vi "main - 副本.vi"() -> ()   [LabVIEW 2017]
uses:
  Ctrl/wave.ctl
  Ctrl/XYGraph.ctl
  <vilib>/Platform/TimedLoop/XDataNode/timing_clust.ctl
  <vilib>/Platform/TimedLoop/XDataNode/nitl_modes.ctl
  <vilib>/Platform/TimedLoop/XDataNode/wakeup.ctl
  <vilib>/Instr/_visa.llb/VISA Configure Serial Port (Instr).vi
  <vilib>/Platform/TimedLoop/XDataNode/XDataNode.xnode
  <vilib>/Platform/TimedLoop/XDataNode/XDNodeRunTimeDep.lvlib
panel:
  out "定时开始":bool=TRUE
  in  "XY缓存":cluster{dbl, dbl}[](array[cluster])
  in  "断开连接时使波形归零":bool
  out "误码":bool
  in  "图表点数":i32
  out "TX":dbl
  out "RX":u64
  in  "连接":bool
  out "串口状态":bool
  in  "波特率":u16(ring) items=["9600", "115200", "256000", "460800", "1000000"]
  in  "端口":string(combo)
  in  "界面切换":enum32{"测控", "后台状态"}(tab)
  in  "Y":enum16{"电流", "电压", "力", "位移", "电阻", "功率", "测试"}(ring)
  in  "X":enum16{"电流", "电压", "力", "位移", "电阻", "功率", "测试"}(ring)
  in  "复位系统":bool
  in  "测量倒计时 S":dbl format="%#.1f"
  out "能量 J":dbl format="%.4g"
  out "质量 g":dbl format="%.3g"
  out "功率 mW":dbl format="%.4g"
  out "电阻 R":dbl format="%.4g"
  in  "自动测量":bool
  out "湿度 %":dbl format="%.2g"
  out "温度 ℃":dbl format="%.2g"
  out "CPU %":u8
  out "位移 mm":dbl format="%.4g"
  out "力 mN":dbl format="%#.2g"
  out "电压 V":dbl format="%.4g"
  out "电流 mA":dbl format="%#.2g"
  in  "校准":bool
  in  "波形归零":bool
  in  "清空图表":bool
  out "持续时间 S":dbl format="%#.2g"
  out "系统时间":string
  in  "发送波形":bool
  out "波形图表":T1
  in  "波形选择":enum32{"斜坡", "正弦", "PWM波", "直流", "控制"}(tab)
  out "斜率k":dbl format="%#.2g"
  in  "通道D":enum16{"DA0", "DA1", "DA01", ""}(ring) caption="通道"
  in  "截距":dbl(slide) min=-5.0 max=5.0 step=0.01 scale=-4.0..4.0
  in  "斜率角":dbl(slide) step=0.01 scale=0.0..180.0
  in  "极值":dbl(slide) min=-5.0 max=5.0 step=0.01 scale=-4.0..4.0
  out "正弦频率":dbl caption="频率 f" format="%#.2g"
  in  "偏距":dbl(slide) min=-5.0 max=5.0 step=0.01 scale=-4.0..4.0
  in  "初相":dbl(slide) min=-6.5 max=6.5 step=0.01 scale=-7.0..7.0
  in  "振幅":dbl(slide) min=0.0 max=5.0 step=0.01 scale=0.0..4.0
  in  "正弦角频率":dbl(slide) caption="角频率" min=0.0 max=100.0 step=0.01 scale=0.0..65.0
  in  "通道S":enum16{"DA0", "DA1", "DA01", ""}(ring) caption="通道"
  in  "通道P":enum16{"DA0", "DA1", "DA01", ""}(ring) caption="通道"
  in  "占空比":dbl(slide) min=0.0 max=1.0 step=0.01 scale=0.0..1.0
  in  "PWM波频率":dbl(slide) caption="频率" min=0.0 max=1000.0 step=0.01 scale=0.0..50.0
  in  "低电压":dbl(slide) min=-5.0 max=5.0 step=0.01 scale=-4.0..4.0
  in  "高电压":dbl(slide) min=-5.0 max=5.0 step=0.01 scale=-4.0..4.0
  in  "DA0":dbl(slide) min=-5.0 max=5.0 step=0.01 scale=-4.0..4.0
  in  "DA1":dbl(slide) min=-5.0 max=5.0 step=0.01 scale=-4.0..4.0
  in  "DA01":dbl(slide) min=-5.0 max=5.0 step=0.01 scale=-4.0..4.0
  in  "控制方法":T2(ring)
  in  "闭环对象":enum16{"位移闭环", "功率闭环", "电流闭环", "力闭环"}(ring)
  in  "外环KP/Bind":dbl
  in  "KD":dbl min=0.0 max=5.0 step=1e-05
  in  "KI / LV":dbl
  in  "发送控制数据":bool
  in  "KP / HV":dbl
  in  "SetPoint":dbl
  in  "控制模式":bool
  in  "板子选择":bool
  out "XY图":T3
  in  "打开图表":bool
  in  "采样率 Hz":u16(ring) items=["10"=10, "20"=20, "50"=50, "100"=100]
  out "定时结束":dbl
  out "匹配剩余":string
  in  "发送区":string
  in  "换行":bool
  in  "send":bool
  in  "清空接收区":bool
  in  "接收间隔ms":u16(ring) items=["50"=50, "100"=100, "150"=150, "200"=200]
  out "实时采样率 Hz":i16
  in  "调试模式":bool
  out "接收区":string
  # "y=kt+b"
  # "y=Asin(ωt+φ)+k"
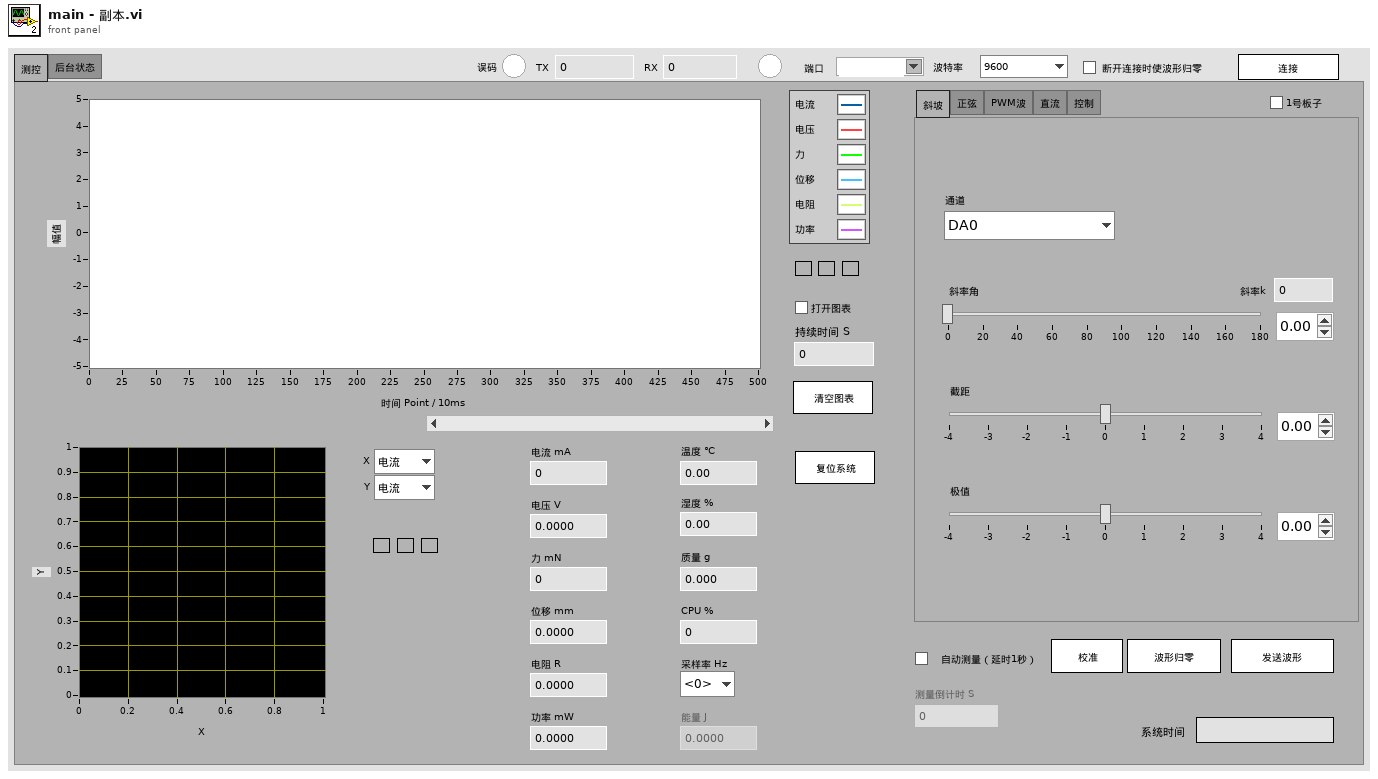
[diagram p1: front panel]
types:
  T1 = typedef "wave.ctl" = cluster{"电流":dbl, "电压":dbl, "力":dbl, "激光":dbl, "电阻":dbl, "功率":dbl}[]
  T2 = enum16{"PID控制", "BangBang控制", "串级PID控制", "自适应控制"}
  T3 = typedef "XYGraph.ctl" = cluster{"X":dbl, "Y":dbl}[]
  T4 = typedef "XDNodeRunTimeDep.lvlib/timing_clust.ctl" = cluster{"Expected End [f-1]":u64, "Actual End [f-1]":u64, "Finished Late? [f-1]":bool, "Expected End [i-1]":u64, "Actual End [i-1]":u64, "Finished Late? [i-1]":bool, "Expected Start [i]":u64, "Actual Start [i]":u64, "Expected Start [f]":u64, "Actual Start [f]":u64, "Source Name":string, "Structure Name":string, "Period":i64, "Deadline":i64, "Offset":i64, "Start":i64, "Priority":i32, "Timeout":i32, "Mode":T5, "Wakeup Reason":T6, "Error":errorcluster, "Source Type":string, "Secondary Source Type":string, "Global End Time":u64, "Global Start Time":u64, "Frame Duration":u64, "Iteration Duration":u64, "Assigned CPU":i32, "I/O Scan Engine Mode":u32}
  T5 = typedef "XDNodeRunTimeDep.lvlib/nitl_modes.ctl" = enum32{"No Change", "Process missed periods, maintain original phase", "Discard missed periods, maintain original phase", "Process missed periods, ignore original phase", "Discard missed periods, ignore original phase"}
  T6 = typedef "XDNodeRunTimeDep.lvlib/wakeup.ctl" = enum32{"Normal", "Aborted", "Asynchronous wakeup", "Timing source error", "Timed loop error", "Timeout"}
  T7 = cluster{"T0时间戳":dbl, "T1时间戳":dbl, "温度":dbl, "湿度":dbl, "CPU使用率":dbl}
  T8 = cluster{"电流":dbl, "电压":dbl, "力":dbl, "激光":dbl, "电阻":dbl, "功率":dbl}[]
  T9 = cluster{"电流":dbl, "电压":dbl, "力":dbl, "激光":dbl, "电阻":dbl, "功率":dbl}
  T10 = cluster{"X":enum16{"电流", "电压", "力", "位移", "电阻", "功率", "测试"}, "Y":enum16{"电流", "电压", "力", "位移", "电阻", "功率", "测试"}}
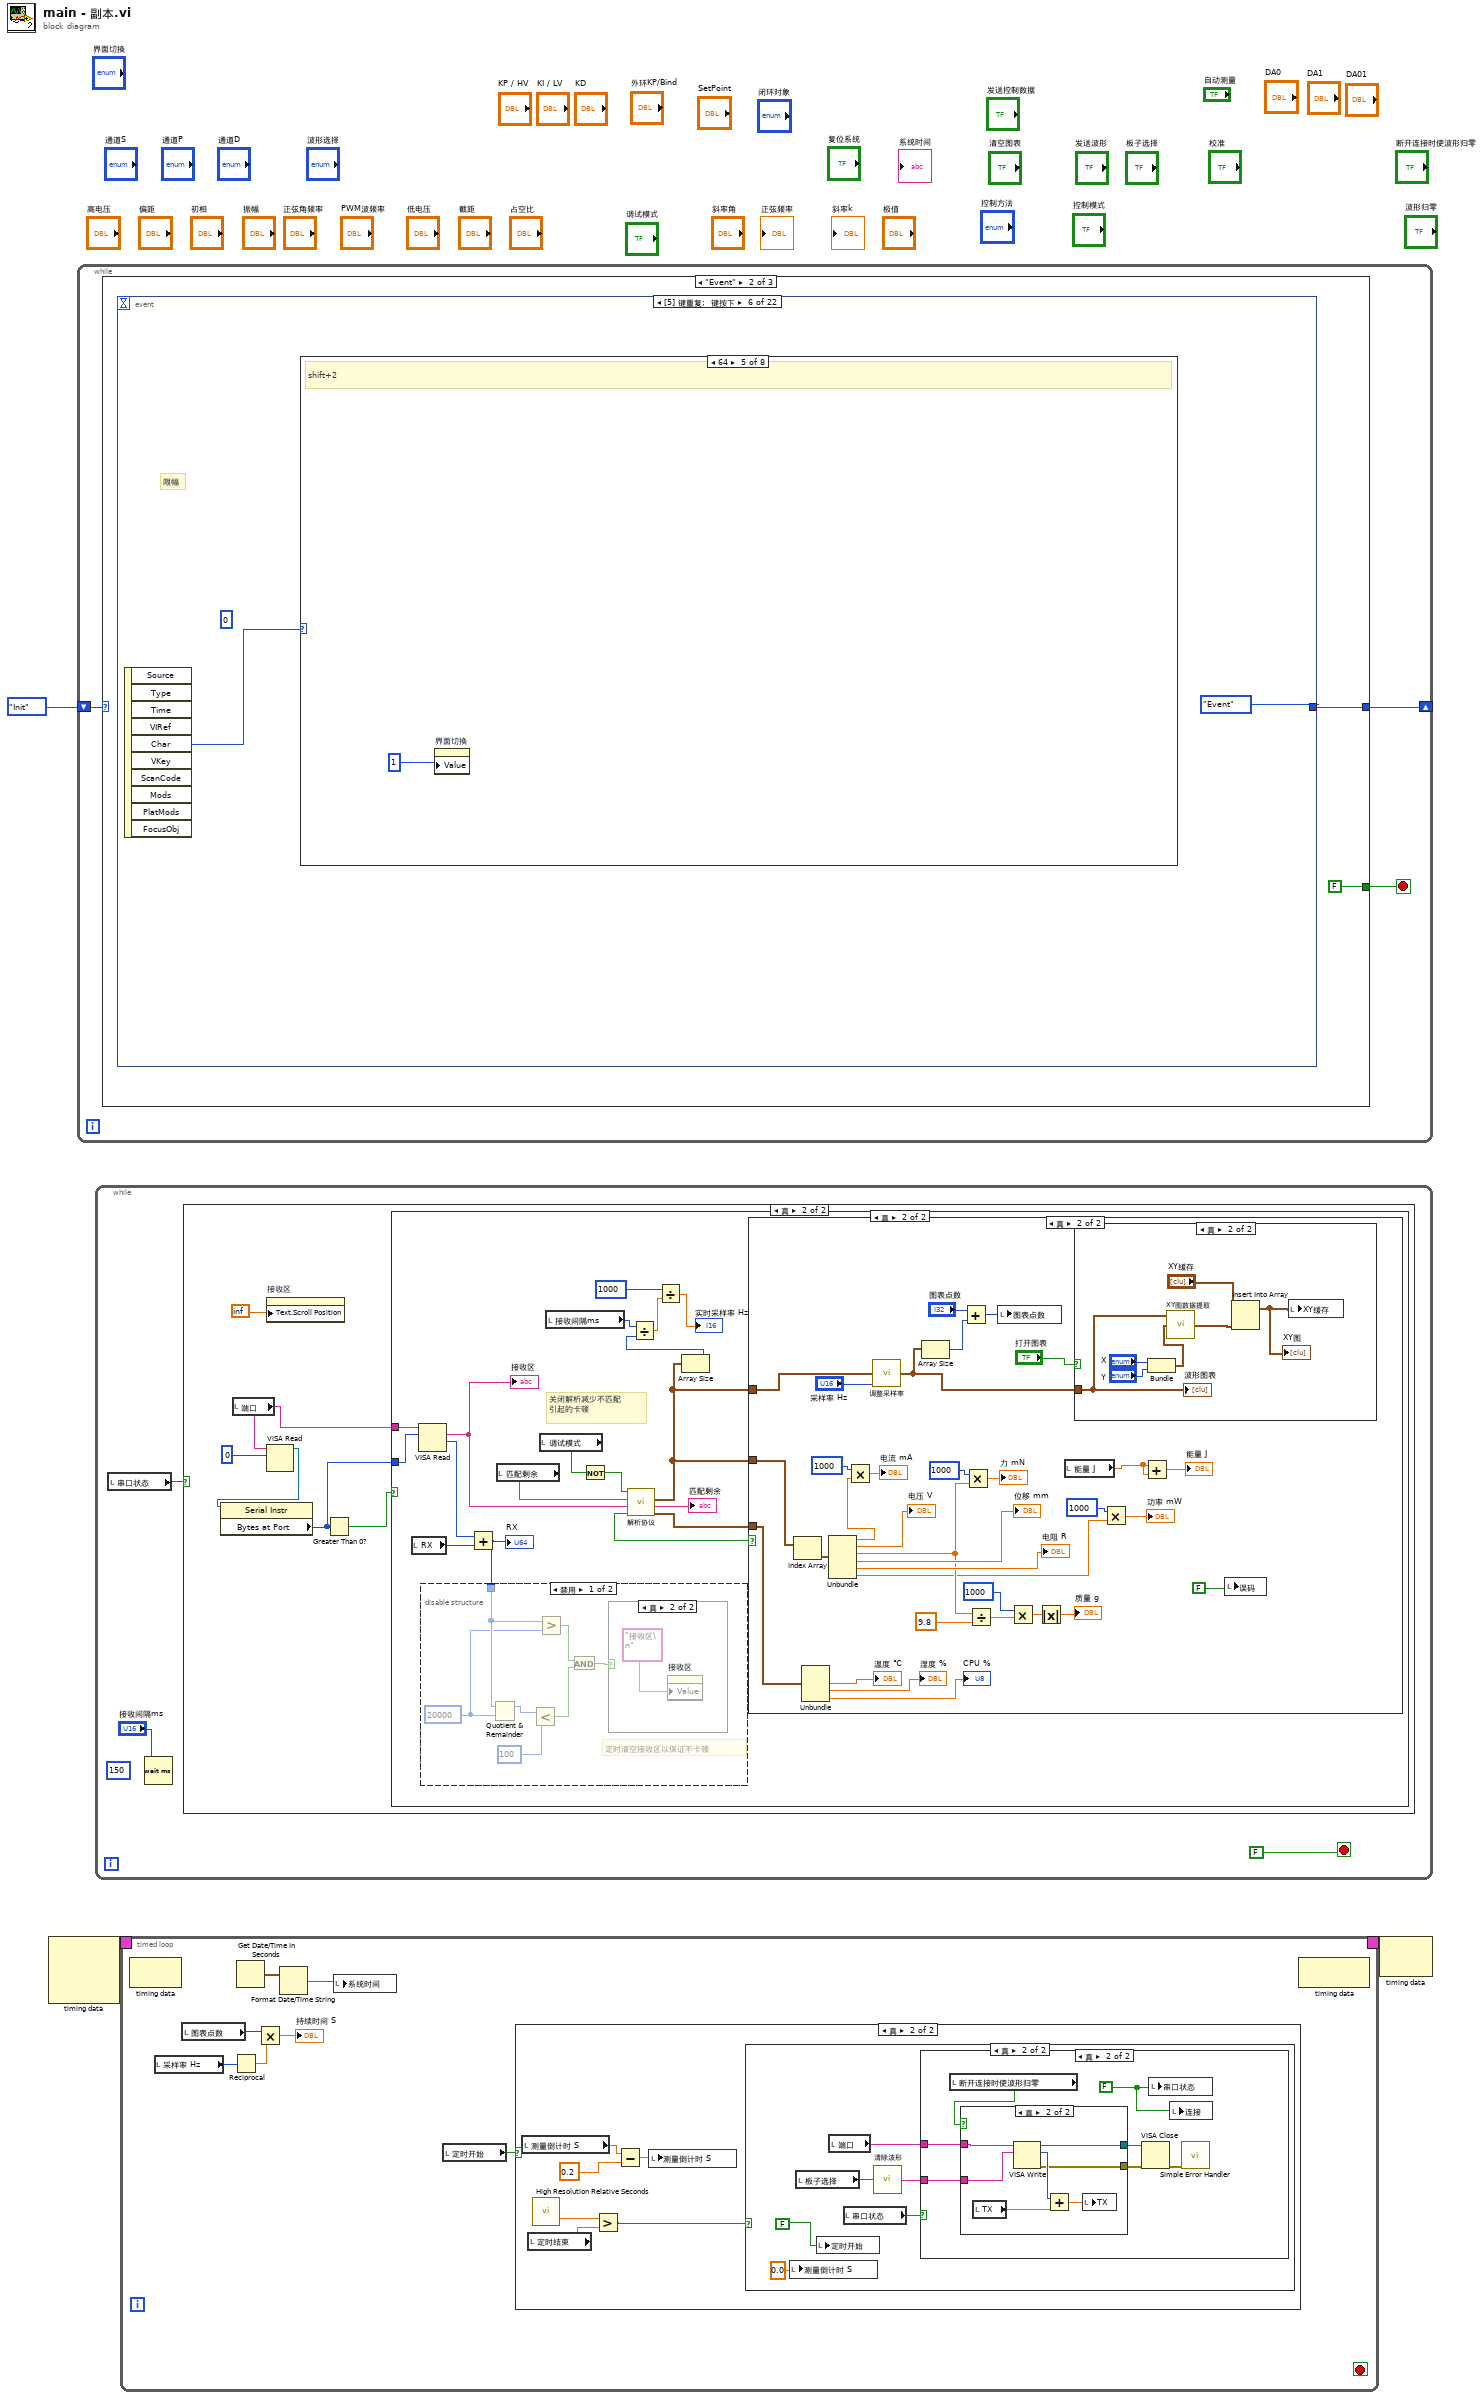
[diagram p0: block diagram]
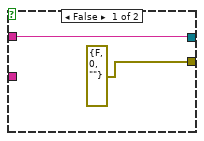
[diagram p5: hidden frame]
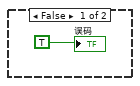
[diagram p10: hidden frame]
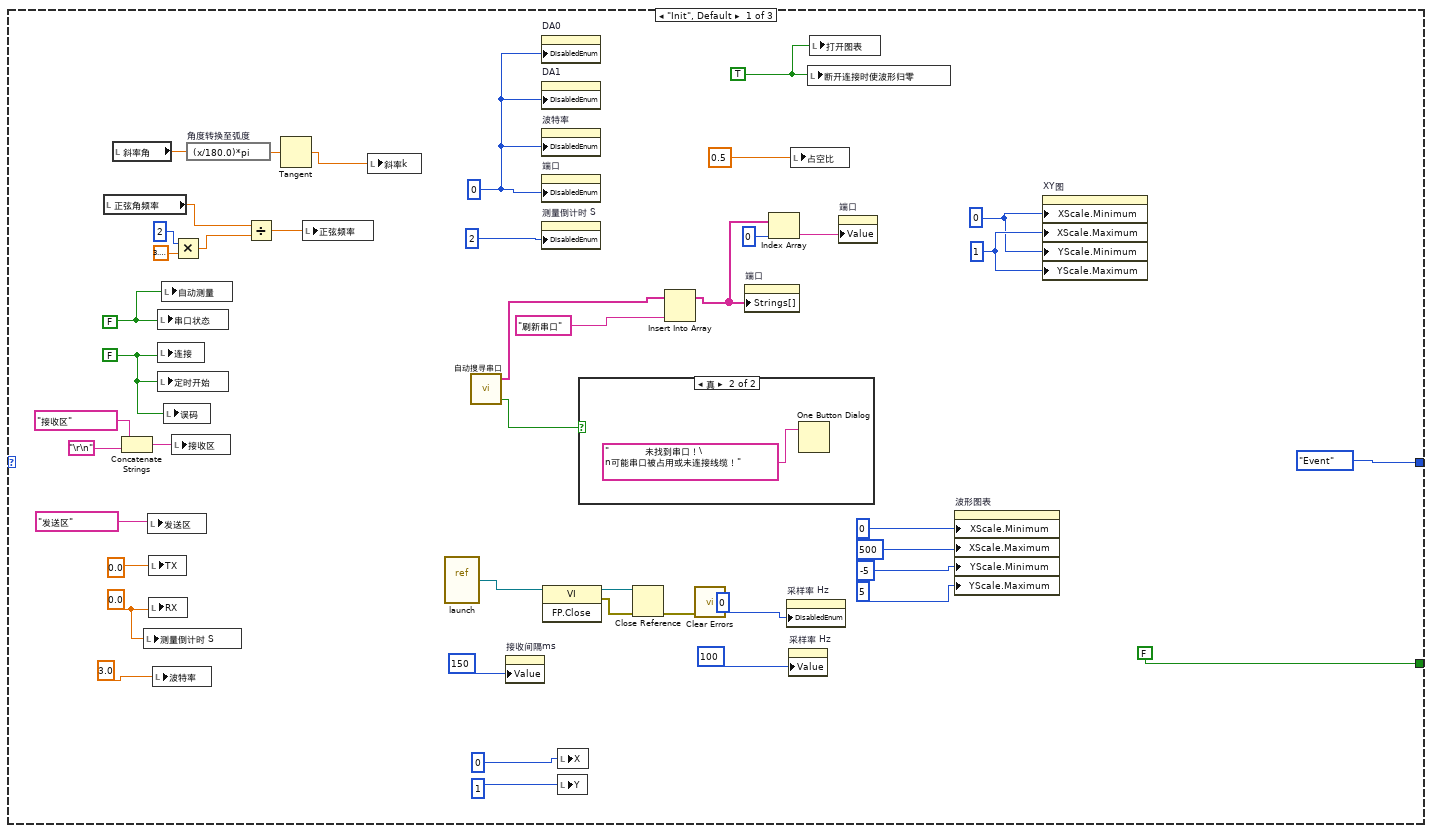
[diagram p12: hidden frame]
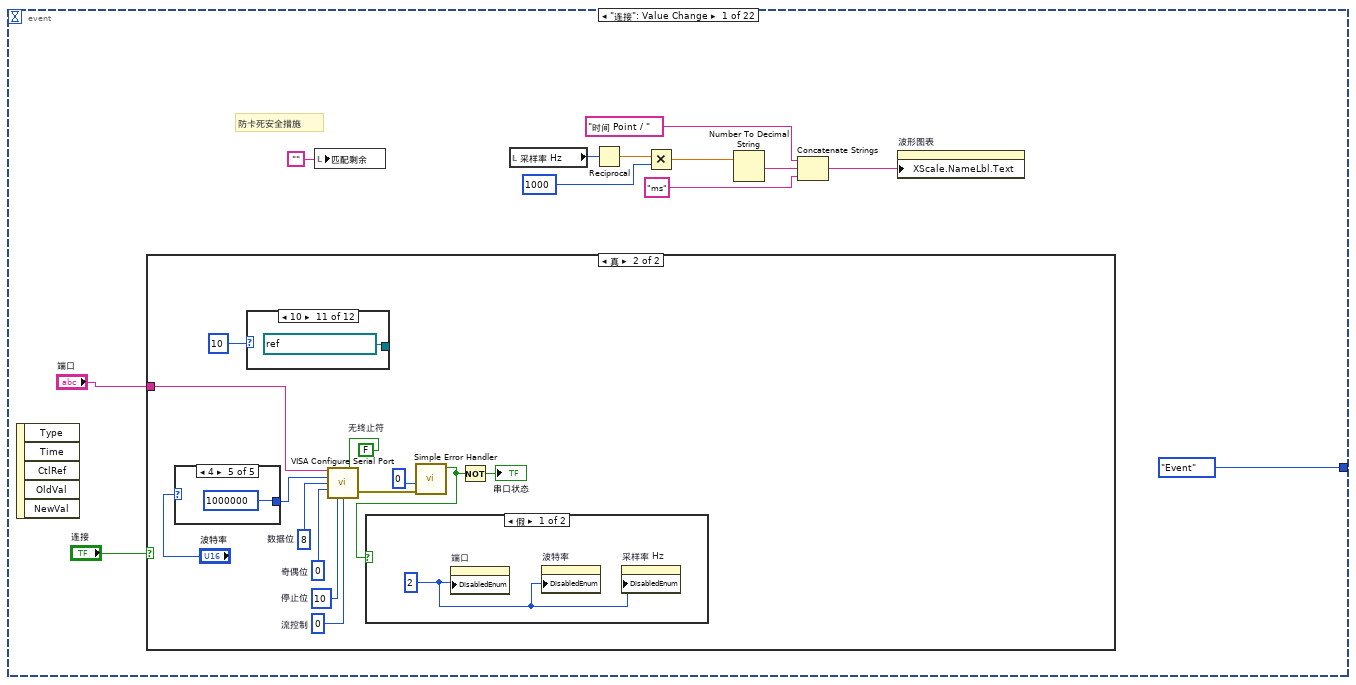
[diagram p14: hidden frame]
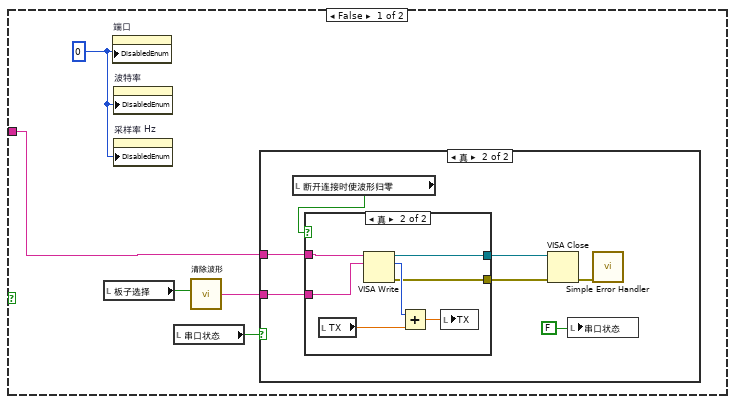
[diagram p15: hidden frame]
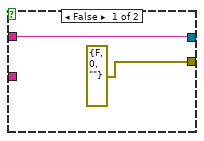
[diagram p17: hidden frame]
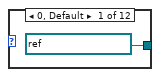
[diagram p18: hidden frame]
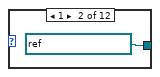
[diagram p19: hidden frame]
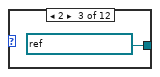
[diagram p20: hidden frame]
diagram:
  n1 = node-c288() -> (w2:T4)  [unwired: 3 in]
  n2 = while {
    shift-right: [w5] -> _
    shift-left: enum16{"Init", "Event", "Exit"}."Init" -> [w6]
    stop <- w4 stop-if-true
    n3 = case shown="\"Event\"" w6 {
      tunnel: [FALSE FALSE TRUE] -> w4
      tunnel: [enum16{"Init", "Event", "Exit"}."Event" w52 enum16{"Init", "Event", "Exit"}."Exit"] -> w5
      frame "Init", Default {
        w13 = 1
        w12 = 0
        w15 = TRUE
        w8 = 0
        w16 = 0.0 ("RX")
        w14 = FALSE
        w11 = FALSE
        n4 = local read "正弦角频率"() -> (w42:dbl)
        n5 = local read "斜率角"() -> (w46:dbl)
        n6 = Concatenate Strings("接收区", "\r\n") -> (w36:string)
        n7 = local write "测量倒计时 S"(w16) -> ()
        n8 = local write "发送区"("发送区") -> ()
        n9 = local write "TX"(0.0 ("TX")) -> ()
        n10 = local write "RX"(w16) -> ()
        n11 = local write "波特率"(3.0 ("RX")) -> ()
        n12 = local write "串口状态"(w14) -> ()
        n13 = local write "连接"(w11) -> ()
        n14 = local write "定时开始"(w11) -> ()
        n15 = local write "自动测量"(w14) -> ()
        n16 = local write "误码"(w11) -> ()
        n17 = local write "接收区"(w36) -> ()
        n18 = Multiply(x=2, y=3.141592653589793) -> (x*y=w41:dbl)
        n19 = expression code="(x/180.0)*pi" "角度转换至弧度"(w46) -> (w47:dbl)
        n20 = Divide(x=w42, y=w41) -> (x/y=w43:dbl)
        n21 = Tangent(1:w47) -> (0:w40:dbl)
        n22 = local write "正弦频率"(w43) -> ()
        n23 = local write "斜率k"(w40) -> ()
        n24 = vi-ref "launch.vi"() -> (w32:refnum<vi>)
        n25 = call "自动搜寻串口.vi"() -> ("找到的串口"=w34:string[], "有错误?"=w35:bool)  [unwired: 6 in, 1 out]
        n26 = property on="接收间隔ms" class="Ring (严格)"("Value"=150) -> ()  [unwired: 2 in, 2 out]
        n27 = property on="DA0" class="Slide (严格)"("DisabledEnum"=w8) -> ()  [unwired: 2 in, 2 out]
        n28 = property on="DA1" class="Slide (严格)"("DisabledEnum"=w8) -> ()  [unwired: 2 in, 2 out]
        n29 = property on="波特率" class="Ring (严格)"("DisabledEnum"=w8) -> ()  [unwired: 2 in, 2 out]
        n30 = property on="端口" class="CmbBox"("DisabledEnum"=w8) -> ()  [unwired: 2 in, 2 out]
        n31 = property on="测量倒计时 S" class="DigNum (严格)"("DisabledEnum"=2) -> ()  [unwired: 2 in, 2 out]
        n32 = invoke class="VI" method="FP.Close"(reference=w32) -> (reference out=w31:refnum<vi>, error out=w30:errorcluster)  [unwired: 2 in, 1 out]
        n33 = local write "X"(0) -> ()
        n34 = local write "Y"(1) -> ()
        n35 = case shown="真" w35 {
          frame False {
          }
          frame True {
            n36 = One Button Dialog(message="            未找到串口！\n可能串口被占用或未连接线缆！") -> ()  [unwired: 1 in, 1 out]
          }
        }
        n37 = Close Reference(reference=w31, error in (no error)=w30) -> (error out=w29:errorcluster)
        n38 = Insert Into Array(array=w34, new element="刷新串口") -> (w28:string[])  [unwired: 1 in]
        n39 = call <vilib>:"Clear Errors.vi"("error in (no error)"=w29) -> ()  [unwired: 5 in, 2 out]
        n40 = property on="端口" class="CmbBox"("Strings[]"=w28) -> ()  [unwired: 2 in, 2 out]
        n41 = Index Array(array=w28, index=0) -> (element=w26:string)
        n42 = property on="采样率 Hz" class="Ring (严格)"("DisabledEnum"=0) -> ()  [unwired: 2 in, 2 out]
        n43 = property on="采样率 Hz" class="Ring (严格)"("Value"=100) -> ()  [unwired: 2 in, 2 out]
        n44 = local write "占空比"(0.5 ("TX")) -> ()
        n45 = local write "断开连接时使波形归零"(w15) -> ()
        n46 = local write "打开图表"(w15) -> ()
        n47 = property on="端口" class="CmbBox"("Value"=w26) -> ()  [unwired: 2 in, 2 out]
        n48 = property on="波形图表" class="WFChart (严格)"("XScale.Minimum"=0, "XScale.Maximum"=500, "YScale.Minimum"=-5, "YScale.Maximum"=5) -> ()  [unwired: 2 in, 2 out]
        n49 = property on="XY图" class="XYGraph (严格)"("XScale.Minimum"=w12, "XScale.Maximum"=w13, "YScale.Minimum"=w12, "YScale.Maximum"=w13) -> ()  [unwired: 2 in, 2 out]
      }
      frame "Event" {
        n50 = event shown="[5] 键重复;  键按下" {
          selector: _ -> [_ _ _ _ _ _ _ _ _ _ _ _ _ _ _ _ _ _ _ _ _ _]
          dyn-events: _ -> [_ _ _ _ _ _ _ _ _ _ _ _ _ _ _ _ _ _ _ _ _ _]
          timeout: _ -> [_ _ _ _ _ _ _ _ _ _ _ _ _ _ _ _ _ _ _ _ _ _]
          tunnel: [enum16{"Init", "Event", "Exit"}."Event" enum16{"Init", "Event", "Exit"}."Event" enum16{"Init", "Event", "Exit"}."Event" enum16{"Init", "Event", "Exit"}."Event" enum16{"Init", "Event", "Exit"}."Event" enum16{"Init", "Event", "Exit"}."Event" enum16{"Init", "Event", "Exit"}."Event" enum16{"Init", "Event", "Exit"}."Event" enum16{"Init", "Event", "Exit"}."Event" enum16{"Init", "Event", "Exit"}."Event" enum16{"Init", "Event", "Exit"}."Event" enum16{"Init", "Event", "Exit"}."Event" enum16{"Init", "Event", "Exit"}."Event" enum16{"Init", "Event", "Exit"}."Event" enum16{"Init", "Event", "Exit"}."Event" enum16{"Init", "Event", "Exit"}."Event" enum16{"Init", "Event", "Exit"}."Event" enum16{"Init", "Event", "Exit"}."Event" enum16{"Init", "Event", "Exit"}."Event" enum16{"Init", "Event", "Exit"}."Event" enum16{"Init", "Event", "Exit"}."Event" enum16{"Init", "Event", "Exit"}."Event"] -> w52
          event "连接": Value Change {
            # "防卡死安全措施"
            n51 = event-data() -> ()  [unwired: 1 in, 5 out]
            n52 = case shown="真" "连接" {
              tunnel: "端口" -> [w66 w87]
              frame False {
                w70 = 0
                n53 = local read "板子选择"() -> (w69:bool)
                n54 = property on="端口" class="CmbBox"("DisabledEnum"=w70) -> ()  [unwired: 2 in, 2 out]
                n55 = property on="波特率" class="Ring (严格)"("DisabledEnum"=w70) -> ()  [unwired: 2 in, 2 out]
                n56 = property on="采样率 Hz" class="Ring (严格)"("DisabledEnum"=w70) -> ()  [unwired: 2 in, 2 out]
                n57 = local read "串口状态"() -> (w68:bool)
                n58 = call "清除波形.vi"("板子选择"=w69) -> ("输出字符串"=w67:string)
                n59 = case shown="真" w68 {
                  tunnel: w67 -> [_ w77]
                  tunnel: w66 -> [_ w72]
                  frame False {
                  }
                  frame True {
                    n60 = local read "断开连接时使波形归零"() -> (w71:bool)
                    n61 = case shown="真" w71 {
                      tunnel: w77 -> [_ w86]
                      tunnel: [w79 w82] -> w74
                      tunnel: [errorcluster {"status"=FALSE, "code"=0, "source"=""} ("错误常量") w81] -> w73
                      tunnel: w72 -> [w79 w80]
                      frame False {
                      }
                      frame True {
                        n62 = local read "TX"() -> (w84:dbl)
                        n63 = VISA Write(VISA resource name=w80, write buffer=w86) -> (VISA resource name out=w82:refnum<visa-resource-name>, return count=w85:u32, error out=w81:errorcluster)  [unwired: 1 in]
                        n64 = Add(x=w85, y=w84) -> (x+y=w83:dbl)
                        n65 = local write "TX"(w83) -> ()
                      }
                    }
                    n66 = VISA Close(VISA resource name=w74, error in (no error)=w73) -> (error out=w75:errorcluster)
                    n67 = local write "串口状态"(FALSE) -> ()
                    n68 = call <vilib>:"Simple Error Handler.vi"("error in (no error)"=w75) -> ()  [unwired: 4 in, 5 out]
                  }
                }
              }
              frame True {
                w90 = FALSE  # 无终止符
                w97 = u16 0  # 流控制
                w96 = u16 10  # 停止位
                w95 = u8 0  # 奇偶位
                w94 = u16 8  # 数据位
                n69 = case shown="4" "波特率" {
                  tunnel: [u32 9600 u32 115200 256000 460800 1000000] -> w93
                  frame 0 {
                  }
                  frame 1, Default {
                  }
                  frame 2 {
                  }
                  frame 3 {
                  }
                  frame 4 {
                  }
                }
                n70 = case shown="10" 10 {
                  tunnel: [refnum<visa-resource-name> "ASRL1::INSTR" ("VISA resource name") refnum<visa-resource-name> "ASRL2::INSTR" ("VISA resource name") refnum<visa-resource-name> "ASRL3::INSTR" ("VISA resource name") refnum<visa-resource-name> "ASRL4::INSTR" ("VISA resource name") refnum<visa-resource-name> "ASRL5::INSTR" ("VISA resource name") refnum<visa-resource-name> "ASRL6::INSTR" ("VISA resource name") refnum<visa-resource-name> "ASRL7::INSTR" ("VISA resource name") refnum<visa-resource-name> "ASRL8::INSTR" ("VISA resource name") refnum<visa-resource-name> "ASRL9::INSTR" ("VISA resource name") refnum<visa-resource-name> "ASRL10::INSTR" ("VISA resource name") refnum<visa-resource-name> "ASRL11::INSTR" ("VISA resource name") refnum<visa-resource-name> "ASRL12::INSTR" ("VISA resource name")] -> _
                  frame 0, Default {
                  }
                  frame 1 {
                  }
                  frame 2 {
                  }
                  frame 3 {
                  }
                  frame 4 {
                  }
                  frame 5 {
                  }
                  frame 6 {
                  }
                  frame 7 {
                  }
                  frame 8 {
                  }
                  frame 9 {
                  }
                  frame 10 {
                  }
                  frame 11 {
                  }
                }
                n71 = call-poly "VISA Configure Serial Port"("VISA resource name"=w87, "Enable Termination\nChar (T)"=w90, "baud rate (9600)"=w93, "data bits (8)"=w94, "parity (0:none)"=w95, "stop bits (10: 1 bit)"=w96, "flow control (0:none)"=w97) -> ("error out"=w98:errorcluster)  [unwired: 7 in, 1 out]
                n72 = call <vilib>:"Simple Error Handler.vi"("type of dialog (OK msg:1)"=0, "error in (no error)"=w98) -> ("error?"=w91:bool)  [unwired: 3 in, 4 out]
                n73 = case shown="假" w91 {
                  frame False {
                    w112 = 2
                    n74 = property on="端口" class="CmbBox"("DisabledEnum"=w112) -> ()  [unwired: 2 in, 2 out]
                    n75 = property on="波特率" class="Ring (严格)"("DisabledEnum"=w112) -> ()  [unwired: 2 in, 2 out]
                    n76 = property on="采样率 Hz" class="Ring (严格)"("DisabledEnum"=w112) -> ()  [unwired: 2 in, 2 out]
                  }
                  frame True {
                    n77 = One Button Dialog(message="串口不存在或已打开！\n请到“设备管理器”查看端口号COM！") -> ()  [unwired: 1 in, 1 out]
                    n78 = local write "连接"(FALSE) -> ()
                  }
                }
                n79 = Not(x=w91) -> (.not. x?=→"串口状态":bool)
              }
            }
            n80 = local write "匹配剩余"("") -> ()
            n81 = local read "采样率 Hz"() -> (w57:u16)
            n82 = Reciprocal(x=w57) -> (1/x=w56:dbl)
            n83 = Multiply(x=w56, y=1000) -> (x*y=w54:dbl)
            n84 = Number To Decimal String(number=w54) -> (decimal integer string=w61:string)  [unwired: 1 in]
            n85 = Concatenate Strings("时间 Point / ", w61, "ms") -> (w60:string)
            n86 = property on="波形图表" class="WFChart (严格)"("XScale.NameLbl.Text"=w60) -> ()  [unwired: 2 in, 2 out]
          }
          event "端口": Value Change {
            n87 = event-data() -> ("NewVal"=w123:string)  [unwired: 1 in, 5 out]
            n88 = Equal?(x=w123, y="刷新串口") -> (x = y?=w121:bool)
            n89 = case shown="真" w121 {
              frame False {
              }
              frame True {
                n90 = call "自动搜寻串口.vi"() -> ("找到的串口"=w127:string[], "有错误?"=w129:bool)  [unwired: 6 in, 1 out]
                n91 = case shown="真" w129 {
                  frame False {
                  }
                  frame True {
                    n92 = One Button Dialog(message="            未找到串口！\n可能串口被占用或未连接线缆！") -> ()  [unwired: 1 in, 1 out]
                  }
                }
                n93 = Insert Into Array(array=w127, new element="刷新串口") -> (w125:string[])  [unwired: 1 in]
                n94 = Index Array(array=w125, index=0) -> (element=w124:string)
                n95 = property on="端口" class="CmbBox"("Strings[]"=w125) -> ()  [unwired: 2 in, 2 out]
                n96 = property on="端口" class="CmbBox"("Value"=w124) -> ()  [unwired: 2 in, 2 out]
              }
            }
          }
          event "send": Mouse Down {
            n97 = event-data() -> ()  [unwired: 1 in, 7 out]
            n98 = local read "串口状态"() -> (w132:bool)
            n99 = case shown="真" w132 {
              frame False {
              }
              frame True {
                n100 = local read "端口"() -> (w133:string)
                n101 = case shown="真" "换行" {
                  tunnel: [_ "\r"] -> w141
                  tunnel: [_ "\n"] -> w140
                  frame False {
                  }
                  frame True {
                  }
                }
                n102 = Concatenate Strings("发送区", w141, w140) -> (w137:string)
                n103 = local read "TX"() -> (w136:dbl)
                n104 = VISA Write(VISA resource name=w133, write buffer=w137) -> (return count=w134:u32)  [unwired: 1 in, 2 out]
                n105 = Add(x=w134, y=w136) -> (x+y=→"TX":dbl)
              }
            }
          }
          event "清空接收区": Mouse Down {
            n106 = event-data() -> ()  [unwired: 1 in, 7 out]
            n107 = local write "接收区"("") -> ()
            n108 = local write "RX"(0.0 ("RX")) -> ()
            n109 = local write "TX"(0.0 ("TX")) -> ()
          }
          event Menu Selection (User) {
            n110 = event-data() -> ("ItemTag"=w148:string)  [unwired: 1 in, 5 out]
            n111 = case shown="\"电路板使用说明\"" w148 {
              frame "关于", Default {
                n112 = call "检查更新.vi"("超时ms"=3000.0) -> ("新版本号"=w152:string)  [unwired: 2 out]
                n113 = call "读取本地版本号.vi"() -> ("版本号"=w159:string)  [unwired: 6 in, 2 out]
                n114 = Concatenate Strings("最新版本号：", w152, "\r\n") -> (w151:string)
                n115 = Concatenate Strings("本地版本号：", w159, "\r\n") -> (w158:string)
                n116 = Concatenate Strings(w151, w158, "By YYH，IBSS，NUAA，NanJing，China") -> (w156:string)
                n117 = One Button Dialog(message=w156) -> ()  [unwired: 1 in, 1 out]
              }
              frame "存储曲线" {
                n118 = One Button Dialog(message="右键图表，点击“导出”即可。\n注意：只能导出显示范围数据，注意缩放") -> ()  [unwired: 1 in, 1 out]
              }
              frame "打开曲线" {
                n119 = One Button Dialog(message="暂不支持") -> ()  [unwired: 1 in, 1 out]
              }
              frame "数据协议" {
                n120 = call <vilib>:"Application Directory.vi"() -> ("Application Directory"=w166:path)
                n121 = call <vilib>:"System Exec.vi"("run minimized? (F)"=TRUE, "wait until completion? (T)"=FALSE, "working directory"=w166, "command line"="cmd /c start protocol.xlsx") -> ("error out"=w167:errorcluster)  [unwired: 4 in, 3 out]
                n122 = call <vilib>:"Simple Error Handler.vi"("error in (no error)"=w167) -> ()  [unwired: 4 in, 5 out]
              }
              frame "电路板使用说明" {
                n123 = One Button Dialog(message="电路板使用说明：\n\n灯光：\n常亮灯：电源指示灯\n闪烁灯：慢闪1次----程序运行正常\n            快闪2次----激光位移传感器通信失败\n            快闪4次----高负载警告\n            颜色--板子编号（蓝LED0、红LED1）\n\n按键：\nKEY键（位于边缘）：切换板子编号。\nRESET键（位于中间）：系统复位。\n\nUSB口：\n用于和电脑连接。\n\nCAN口：\n用于多电路板连接，CANH连CANH，CANL连CANL，并保证闪烁的灯颜色不一致。\n\nRJ11口（RS232）：\n用于和激光位移传感器KEYENCE LKGD500连接。") -> ()  [unwired: 1 in, 1 out]
              }
              frame "上位机使用说明" {
                n124 = One Button Dialog(message="上位机使用说明：\n\n鼠标悬停在部分控件上会自动出现说明提示。\n\nlaunch.exe：\n该文件为启动文件，用于检查软件更新，由于GitHub偶尔访问较慢，可进安装目录直接运行IPMC.exe（主程序文件）。\n\n连接：\n选择“端口号（刷新串口）”、“波特率（460800）”，点击“连接”--建立通信。\n\n误码：红灯亮起表示数据解析异常，请等待或重新连接。\n\n1/2号板子：\n选择要控制的电路板，1号板子--蓝灯闪烁，2号板子--红灯闪烁。\n\n快捷键：\n规划中...\n\n图表：\n1. 右键图表可以勾选自动缩放、存储曲线等功能；\n2. 导出曲线只导出可见范围内数据，要导出所有数据请先调整标尺；\n3. 图表缓存大小：1048576点；") -> ()  [unwired: 1 in, 1 out]
              }
            }
          }
          event Key Repeat; Key Down {
            (unwired) 0
            # "限幅"
            n125 = event-data() -> ("Char"=w170:i16)  [unwired: 1 in, 9 out]
            n126 = case "条件结构" shown="64" w170 {
              frame 0, Default {
              }
              frame 32 {
                # "空格"
                n127 = disable-structure shown="禁用" {
                  frame Disabled {
                    n128 = local read "板子选择"() -> (w173:bool)
                    n129 = local read "波形选择"() -> (w176:enum32{"斜坡", "正弦", "PWM波", "直流", "控制"})
                    n130 = Boolean To (0,1)(Boolean=w173) -> (0, 1=w172:i16)
                    n131 = case shown="\"斜坡\", 默认" w176 {
                      selector: w176 -> [w186 w199 w214 _]
                      tunnel: [w193 w202 w217 "\r\n"] -> w174
                      tunnel: w172 -> [w185 w198 w213 _]
                      frame "斜坡", Default {
                        w197 = 170
                        n132 = local read "通道D"() -> (w187:enum16{"DA0", "DA1", "DA01", ""})
                        n133 = local read "斜率k"() -> (w192:dbl)
                        n134 = local read "极值"() -> (w190:dbl)
                        n135 = local read "截距"() -> (w195:dbl)
                        n136 = call "浮点转字节数组.vi"("输入"=w190) -> ("数组，高字节在前"=w188:u8[])  [unwired: 3 in, 4 out]
                        n137 = call "浮点转字节数组.vi"("输入"=w192) -> ("数组，高字节在前"=w196:u8[])  [unwired: 3 in, 4 out]
                        n138 = call "浮点转字节数组.vi"("输入"=w195) -> ("数组，高字节在前"=w194:u8[])  [unwired: 3 in, 4 out]
                        n139 = Build Array (concatenate)(w197, w197, w185, w187, w186, w196, w194, w188, 0) -> (w191:u32[])
                        n140 = Byte Array To String(unsigned byte array=w191) -> (string=w193:string)
                        n141 = local write "发送区"(w193) -> ()
                      }
                      frame "正弦" {
                        w212 = 170
                        n142 = local read "通道S"() -> (w200:enum16{"DA0", "DA1", "DA01", ""})
                        n143 = local read "正弦角频率"() -> (w209:dbl)
                        n144 = local read "初相"() -> (w208:dbl)
                        n145 = local read "偏距"() -> (w204:dbl)
                        n146 = local read "振幅"() -> (w211:dbl)
                        n147 = call "浮点转字节数组.vi"("输入"=w211) -> ("数组，高字节在前"=w210:u8[])  [unwired: 3 in, 4 out]
                        n148 = call "浮点转字节数组.vi"("输入"=w209) -> ("数组，高字节在前"=w207:u8[])  [unwired: 3 in, 4 out]
                        n149 = call "浮点转字节数组.vi"("输入"=w208) -> ("数组，高字节在前"=w206:u8[])  [unwired: 3 in, 4 out]
                        n150 = call "浮点转字节数组.vi"("输入"=w204) -> ("数组，高字节在前"=w205:u8[])  [unwired: 3 in, 4 out]
                        n151 = Build Array (concatenate)(w212, w212, w198, w200, w199, w210, w207, w206, w205, 0) -> (w201:u32[])
                        n152 = Byte Array To String(unsigned byte array=w201) -> (string=w202:string)
                        n153 = local write "发送区"(w202) -> ()
                      }
                      frame "PWM波" {
                        w227 = 170
                        n154 = local read "通道P"() -> (w215:enum16{"DA0", "DA1", "DA01", ""})
                        n155 = local read "PWM波频率"() -> (w222:dbl)
                        n156 = local read "占空比"() -> (w220:dbl)
                        n157 = local read "高电压"() -> (w226:dbl)
                        n158 = local read "低电压"() -> (w224:dbl)
                        n159 = call "浮点转字节数组.vi"("输入"=w226) -> ("数组，高字节在前"=w225:u8[])  [unwired: 3 in, 4 out]
                        n160 = call "浮点转字节数组.vi"("输入"=w224) -> ("数组，高字节在前"=w223:u8[])  [unwired: 3 in, 4 out]
                        n161 = call "浮点转字节数组.vi"("输入"=w222) -> ("数组，高字节在前"=w221:u8[])  [unwired: 3 in, 4 out]
                        n162 = call "浮点转字节数组.vi"("输入"=w220) -> ("数组，高字节在前"=w219:u8[])  [unwired: 3 in, 4 out]
                        n163 = Build Array (concatenate)(w227, w227, w213, w215, w214, w225, w223, w221, w219, 0) -> (w216:u32[])
                        n164 = Byte Array To String(unsigned byte array=w216) -> (string=w217:string)
                        n165 = local write "发送区"(w217) -> ()
                      }
                      frame "直流" {
                      }
                    }
                    n166 = local read "串口状态"() -> (w175:bool)
                    n167 = case shown="真" w175 {
                      tunnel: w174 -> [_ w179]
                      frame False {
                        n168 = One Button Dialog(message="未连接平台！") -> ()  [unwired: 1 in, 1 out]
                      }
                      frame True {
                        n169 = local read "端口"() -> (w178:string)
                        n170 = Concatenate Strings(w179, "\r\n") -> (w184:string)
                        n171 = local read "TX"() -> (w182:dbl)
                        n172 = VISA Write(VISA resource name=w178, write buffer=w184) -> (return count=w183:u32)  [unwired: 1 in, 2 out]
                        n173 = Add(x=w183, y=w182) -> (x+y=w180:dbl)
                        n174 = local write "TX"(w180) -> ()
                      }
                    }
                  }
                  frame Enabled {
                  }
                }
              }
              frame 48 {
                # "字符0"
                n175 = disable-structure shown="禁用" {
                  frame Disabled {
                    w231 = 3  # 类型强制直流
                    w229 = 0.0
                    w232 = 2  # 通道
                    w233 = 170
                    n176 = local read "板子选择"() -> (w235:bool)
                    n177 = Boolean To (0,1)(Boolean=w235) -> (0, 1=w234:i16)
                    n178 = call "浮点转字节数组.vi"("输入"=w229) -> ("数组，高字节在前"=w236:u8[])  [unwired: 3 in, 4 out]
                    n179 = local write "DA0"(w229) -> ()
                    n180 = local write "DA1"(w229) -> ()
                    n181 = Build Array (concatenate)(w233, w233, w234, w232, w231, w236, w236, 0) -> (w239:i32[])
                    n182 = Byte Array To String(unsigned byte array=w239) -> (string=w238:string)
                    n183 = local write "发送区"(w238) -> ()
                    n184 = local read "串口状态"() -> (w237:bool)
                    n185 = case shown="真" w237 {
                      tunnel: w238 -> [_ w242]
                      frame False {
                        n186 = One Button Dialog(message="未连接平台！") -> ()  [unwired: 1 in, 1 out]
                      }
                      frame True {
                        n187 = local read "端口"() -> (w241:string)
                        n188 = Concatenate Strings(w242, "\r\n") -> (w247:string)
                        n189 = VISA Write(VISA resource name=w241, write buffer=w247) -> (return count=w246:u32)  [unwired: 1 in, 2 out]
                        n190 = local read "TX"() -> (w245:dbl)
                        n191 = Add(x=w246, y=w245) -> (x+y=w243:dbl)
                        n192 = local write "TX"(w243) -> ()
                      }
                    }
                  }
                  frame Enabled {
                  }
                }
              }
              frame 33 {
                # "shift+1"
                n193 = disable-structure shown="禁用" {
                  frame Disabled {
                    w256 = 1  # 通道
                    w261 = 170
                    n194 = local read "DA1"() -> (w264:dbl)
                    n195 = Add(x=-0.1, y=w264) -> (x+y=w262:dbl)
                    n196 = local write "DA1"(w262) -> ()
                    n197 = local read "板子选择"() -> (w255:bool)
                    n198 = local read "DA1"() -> (w252:dbl)
                    n199 = local read "DA0"() -> (w253:dbl)
                    n200 = Boolean To (0,1)(Boolean=w255) -> (0, 1=w254:i16)
                    n201 = call "浮点转字节数组.vi"("输入"=w253) -> ("数组，高字节在前"=w260:u8[])  [unwired: 3 in, 4 out]
                    n202 = call "浮点转字节数组.vi"("输入"=w252) -> ("数组，高字节在前"=w259:u8[])  [unwired: 3 in, 4 out]
                    n203 = Build Array (concatenate)(w261, w261, w254, w256, 3, w260, w259, 0) -> (w257:i32[])
                    n204 = local read "串口状态"() -> (w251:bool)
                    n205 = Byte Array To String(unsigned byte array=w257) -> (string=w250:string)
                    n206 = case shown="真" w251 {
                      tunnel: w250 -> [_ w269]
                      frame False {
                      }
                      frame True {
                        n207 = local read "端口"() -> (w271:string)
                        n208 = Concatenate Strings(w269, "\r\n") -> (w268:string)
                        n209 = local read "TX"() -> (w267:dbl)
                        n210 = VISA Write(VISA resource name=w271, write buffer=w268) -> (return count=w266:u32)  [unwired: 1 in, 2 out]
                        n211 = Add(x=w266, y=w267) -> (x+y=w265:dbl)
                        n212 = local write "TX"(w265) -> ()
                      }
                    }
                  }
                  frame Enabled {
                  }
                }
                n213 = property on="界面切换" class="TabCtl (严格)"("Value"=0) -> ()  [unwired: 2 in, 2 out]
              }
              frame 64 {
                # "shift+2"
                n214 = property on="界面切换" class="TabCtl (严格)"("Value"=1) -> ()  [unwired: 2 in, 2 out]
              }
              frame 51 {
                # "字符3"
                n215 = disable-structure shown="禁用" {
                  frame Disabled {
                    w279 = 1  # 通道
                    w281 = 170
                    n216 = local read "DA1"() -> (w288:dbl)
                    n217 = Add(x=0.1, y=w288) -> (x+y=w286:dbl)
                    n218 = local write "DA1"(w286) -> ()
                    n219 = local read "板子选择"() -> (w280:bool)
                    n220 = local read "DA0"() -> (w278:dbl)
                    n221 = local read "DA1"() -> (w277:dbl)
                    n222 = Boolean To (0,1)(Boolean=w280) -> (0, 1=w282:i16)
                    n223 = call "浮点转字节数组.vi"("输入"=w278) -> ("数组，高字节在前"=w285:u8[])  [unwired: 3 in, 4 out]
                    n224 = call "浮点转字节数组.vi"("输入"=w277) -> ("数组，高字节在前"=w284:u8[])  [unwired: 3 in, 4 out]
                    n225 = Build Array (concatenate)(w281, w281, w282, w279, 3, w285, w284, 0) -> (w275:i32[])
                    n226 = local read "串口状态"() -> (w276:bool)
                    n227 = Byte Array To String(unsigned byte array=w275) -> (string=w274:string)
                    n228 = case shown="真" w276 {
                      tunnel: w274 -> [_ w295]
                      frame False {
                      }
                      frame True {
                        n229 = local read "端口"() -> (w292:string)
                        n230 = Concatenate Strings(w295, "\r\n") -> (w293:string)
                        n231 = local read "TX"() -> (w290:dbl)
                        n232 = VISA Write(VISA resource name=w292, write buffer=w293) -> (return count=w289:u32)  [unwired: 1 in, 2 out]
                        n233 = Add(x=w289, y=w290) -> (x+y=w291:dbl)
                        n234 = local write "TX"(w291) -> ()
                      }
                    }
                  }
                  frame Enabled {
                  }
                }
              }
              frame 52 {
                # "字符4"
                n235 = disable-structure shown="禁用" {
                  frame Disabled {
                    w307 = 0  # 通道
                    w311 = 170
                    n236 = local read "DA0"() -> (w305:dbl)
                    n237 = Add(x=-0.1, y=w305) -> (x+y=w303:dbl)
                    n238 = local write "DA0"(w303) -> ()
                    n239 = local read "板子选择"() -> (w302:bool)
                    n240 = local read "DA1"() -> (w300:dbl)
                    n241 = local read "DA0"() -> (w301:dbl)
                    n242 = Boolean To (0,1)(Boolean=w302) -> (0, 1=w306:i16)
                    n243 = call "浮点转字节数组.vi"("输入"=w301) -> ("数组，高字节在前"=w310:u8[])  [unwired: 3 in, 4 out]
                    n244 = call "浮点转字节数组.vi"("输入"=w300) -> ("数组，高字节在前"=w309:u8[])  [unwired: 3 in, 4 out]
                    n245 = Build Array (concatenate)(w311, w311, w306, w307, 3, w310, w309, 0) -> (w299:i32[])
                    n246 = local read "串口状态"() -> (w297:bool)
                    n247 = Byte Array To String(unsigned byte array=w299) -> (string=w298:string)
                    n248 = case shown="真" w297 {
                      tunnel: w298 -> [_ w318]
                      frame False {
                      }
                      frame True {
                        n249 = local read "端口"() -> (w315:string)
                        n250 = Concatenate Strings(w318, "\r\n") -> (w316:string)
                        n251 = VISA Write(VISA resource name=w315, write buffer=w316) -> (return count=w314:u32)  [unwired: 1 in, 2 out]
                        n252 = local read "TX"() -> (w313:dbl)
                        n253 = Add(x=w314, y=w313) -> (x+y=w312:dbl)
                        n254 = local write "TX"(w312) -> ()
                      }
                    }
                  }
                  frame Enabled {
                  }
                }
              }
              frame 54 {
                # "字符6"
                n255 = disable-structure shown="禁用" {
                  frame Disabled {
                    w330 = 0  # 通道
                    w334 = 170
                    n256 = local read "DA0"() -> (w328:dbl)
                    n257 = Add(x=0.1, y=w328) -> (x+y=w327:dbl)
                    n258 = local write "DA0"(w327) -> ()
                    n259 = local read "板子选择"() -> (w325:bool)
                    n260 = local read "DA0"() -> (w324:dbl)
                    n261 = local read "DA0"() -> (w323:dbl)
                    n262 = Boolean To (0,1)(Boolean=w325) -> (0, 1=w329:i16)
                    n263 = call "浮点转字节数组.vi"("输入"=w324) -> ("数组，高字节在前"=w333:u8[])  [unwired: 3 in, 4 out]
                    n264 = call "浮点转字节数组.vi"("输入"=w323) -> ("数组，高字节在前"=w332:u8[])  [unwired: 3 in, 4 out]
                    n265 = Build Array (concatenate)(w334, w334, w329, w330, 3, w333, w332, 0) -> (w322:i32[])
                    n266 = local read "串口状态"() -> (w320:bool)
                    n267 = Byte Array To String(unsigned byte array=w322) -> (string=w321:string)
                    n268 = case shown="假" w320 {
                      tunnel: w321 -> [_ w341]
                      frame False {
                      }
                      frame True {
                        n269 = Concatenate Strings(w341, "\r\n") -> (w339:string)
                        n270 = local read "端口"() -> (w338:string)
                        n271 = VISA Write(VISA resource name=w338, write buffer=w339) -> (return count=w337:u32)  [unwired: 1 in, 2 out]
                        n272 = local read "TX"() -> (w336:dbl)
                        n273 = Add(x=w337, y=w336) -> (x+y=w335:dbl)
                        n274 = local write "TX"(w335) -> ()
                      }
                    }
                  }
                  frame Enabled {
                  }
                }
              }
            }
          }
          event "清空图表": Mouse Up {
            n275 = event-data() -> ()  [unwired: 1 in, 8 out]
            n276 = Two Button Dialog(message="确认清空图表吗？") -> (T button?=w342:bool)  [unwired: 2 in]
            n277 = case shown="真" w342 {
              frame False {
              }
              frame True {
                w350 = 1
                w351 = 0
                w352 = cluster{dbl, dbl}[] []
                w349 = 0
                n278 = local write "图表点数"(w349) -> ()
                n279 = property on="波形图表" class="WFChart (严格)"("XScale.Minimum"=w349, "XScale.Maximum"=500, "YScale.Minimum"=-5, "YScale.Maximum"=5) -> ()  [unwired: 2 in, 2 out]
                n280 = local write "XY缓存"(w352) -> ()
                n281 = property on="XY图" class="XYGraph (严格)"("Value"=w352) -> ()  [unwired: 2 in, 2 out]
                n282 = property on="波形图表" class="WFChart (严格)"("History Data"=cluster{dbl, dbl, dbl, dbl, dbl, dbl}[] []) -> ()  [unwired: 2 in, 2 out]
                n283 = property on="XY图" class="XYGraph (严格)"("XScale.Minimum"=w351, "XScale.Maximum"=w350, "YScale.Minimum"=w351, "YScale.Maximum"=w350) -> ()  [unwired: 2 in, 2 out]
              }
            }
          }
          event "X", "Y": Value Change {
            w353 = cluster{dbl, dbl}[] []
            n284 = event-data() -> ()  [unwired: 1 in, 6 out]
            n285 = local write "XY缓存"(w353) -> ()
            n286 = property on="XY图" class="XYGraph (严格)"("Value"=w353) -> ()  [unwired: 2 in, 2 out]
          }
          event "校准": Mouse Up {
            w355 = u16 170 items=["0xAA"=170, "CH0"=0, "CH1"=1, "CH01"=2, "CARLIB"=85, "SWITCH"=86, "CONTROL"=87]
            w356 = u16 85 items=["0xAA"=170, "CH0"=0, "CH1"=1, "CH01"=2, "CARLIB"=85, "SWITCH"=86, "CONTROL"=87]
            w359 = "\r\n"
            n287 = event-data() -> ()  [unwired: 1 in, 8 out]
            n288 = local read "板子选择"() -> (w365:bool)
            n289 = Boolean To (0,1)(Boolean=w365) -> (0, 1=w364:i16)
            n290 = Build Array(w355, w355, w364, w356, w356) -> (w363:u16[])
            n291 = Byte Array To String(unsigned byte array=w363) -> (string=w362:string)
            n292 = Concatenate Strings(w362, "CARLIB", w359, w359) -> (w357:string)
            n293 = local read "串口状态"() -> (w361:bool)
            n294 = local write "发送区"(w357) -> ()
            n295 = case shown="真" w361 {
              tunnel: w357 -> [_ w366]
              frame False {
              }
              frame True {
                n296 = local read "端口"() -> (w368:string)
                n297 = local read "TX"() -> (w369:dbl)
                n298 = VISA Write(VISA resource name=w368, write buffer=w366) -> (return count=w367:u32)  [unwired: 1 in, 2 out]
                n299 = Add(x=w367, y=w369) -> (x+y=w370:dbl)
                n300 = local write "TX"(w370) -> ()
              }
            }
          }
          event "波形归零": Mouse Up; "控制模式", "调试模式": Value Change {
            w381 = u16 170 items=["0xAA"=170, "CH0"=0, "CH1"=1, "CH01"=2, "CARLIB"=85, "SWITCH"=86, "CONTROL"=87]
            w380 = u16 86 items=["0xAA"=170, "CH0"=0, "CH1"=1, "CH01"=2, "CARLIB"=85, "SWITCH"=86, "CONTROL"=87]
            n301 = event-data() -> ()  [unwired: 1 in, 4 out]
            n302 = local read "控制模式"() -> (w379:bool)
            n303 = local read "板子选择"() -> (w383:bool)
            n304 = case shown="假" w379 {
              tunnel: 0 -> [w394 w398]
              tunnel: [w393 w396] -> w376
              frame False {
                n305 = And(x=127, y=w394) -> (x .and. y?=w393:i32)
              }
              frame True {
                n306 = Or(x=128, y=w398) -> (x .or. y?=w396:i32)
              }
            }
            n307 = Boolean To (0,1)(Boolean=w383) -> (0, 1=w382:i16)
            n308 = local read "串口状态"() -> (w385:bool)
            n309 = call "清除波形.vi"() -> ()  [unwired: 1 in, 1 out]
            n310 = local read "调试模式"() -> (w377:bool)
            n311 = case shown="真" w377 {
              tunnel: w376 -> [w388 w392]
              tunnel: [w387 w390] -> w375
              frame False {
                n312 = And(x=191, y=w388) -> (x .and. y?=w387:i32)
              }
              frame True {
                n313 = Or(x=64, y=w392) -> (x .or. y?=w390:i32)
              }
            }
            n314 = Or(x=32, y=w375) -> (x .or. y?=w373:i32)
            n315 = Build Array(w381, w381, w382, w380, w380, w373, 0) -> (w384:i32[])
            n316 = Byte Array To String(unsigned byte array=w384) -> (string=w371:string)
            n317 = case shown="真" w385 {
              tunnel: w371 -> [_ w401]
              frame False {
                n318 = One Button Dialog(message="未连接平台！") -> ()  [unwired: 1 in, 1 out]
              }
              frame True {
                w400 = 0.0
                n319 = local read "端口"() -> (w402:string)
                n320 = local read "TX"() -> (w404:dbl)
                n321 = VISA Write(VISA resource name=w402, write buffer=w401) -> (return count=w405:u32)  [unwired: 1 in, 2 out]
                n322 = Add(x=w405, y=w404) -> (x+y=w403:dbl)
                n323 = local write "DA0"(w400) -> ()
                n324 = local write "DA1"(w400) -> ()
                n325 = local write "DA01"(w400) -> ()
                n326 = local write "TX"(w403) -> ()
              }
            }
          }
          event "复位系统": Mouse Up {
            n327 = event-data() -> ()  [unwired: 1 in, 8 out]
            n328 = Two Button Dialog(message="确认复位电路板吗？") -> (T button?=w407:bool)  [unwired: 2 in]
            n329 = case shown="真" w407 {
              frame False {
              }
              frame True {
                w416 = u16 170 items=["0xAA"=170, "CH0"=0, "CH1"=1, "CH01"=2, "CARLIB"=85, "SWITCH"=86, "CONTROL"=87]
                w417 = u16 86 items=["0xAA"=170, "CH0"=0, "CH1"=1, "CH01"=2, "CARLIB"=85, "SWITCH"=86, "CONTROL"=87]
                n330 = local read "板子选择"() -> (w415:bool)
                n331 = Boolean To (0,1)(Boolean=w415) -> (0, 1=w414:i16)
                n332 = local read "串口状态"() -> (w411:bool)
                n333 = Build Array(w416, w416, w414, w417, w417, 8, 0) -> (w412:i32[])
                n334 = Byte Array To String(unsigned byte array=w412) -> (string=w410:string)
                n335 = case shown="真" w411 {
                  tunnel: w410 -> [_ w419]
                  frame False {
                    n336 = One Button Dialog(message="未连接平台！") -> ()  [unwired: 1 in, 1 out]
                  }
                  frame True {
                    n337 = local read "端口"() -> (w423:string)
                    n338 = local read "TX"() -> (w422:dbl)
                    n339 = VISA Write(VISA resource name=w423, write buffer=w419) -> (return count=w420:u32)  [unwired: 1 in, 2 out]
                    n340 = Add(x=w420, y=w422) -> (x+y=w421:dbl)
                    n341 = local write "TX"(w421) -> ()
                  }
                }
              }
            }
          }
          event "发送波形": Mouse Up {
            n342 = event-data() -> ()  [unwired: 1 in, 8 out]
            n343 = flat-sequence {
              frame #0 {
                n344 = local read "自动测量"() -> (w425:bool)
                n345 = case shown="真" w425 {
                  frame False {
                  }
                  frame True {
                    w430 = 1
                    w431 = 0
                    w429 = 0
                    w435 = cluster{dbl, dbl}[] []
                    n346 = local write "图表点数"(w429) -> ()
                    n347 = Greater Than 0?(x="测量倒计时 S") -> (x > 0?=w432:bool)
                    n348 = property on="波形图表" class="WFChart (严格)"("XScale.Minimum"=w429, "XScale.Maximum"=500, "YScale.Minimum"=-5, "YScale.Maximum"=5) -> ()  [unwired: 2 in, 2 out]
                    n349 = case shown="真" w432 {
                      frame False {
                      }
                      frame True {
                        n350 = local read "测量倒计时 S"() -> (w440:dbl)
                        n351 = call <vilib>:"High Resolution Relative Seconds.vi"() -> ("relative seconds"=w441:dbl)
                        n352 = Add(x=w441, y=w440) -> (x+y=→"定时结束":dbl)
                        "定时开始" <- TRUE
                      }
                    }
                    n353 = local write "图表点数"(0.0) -> ()
                    n354 = local write "XY缓存"(w435) -> ()
                    n355 = property on="波形图表" class="WFChart (严格)"("History Data"=cluster{dbl, dbl, dbl, dbl, dbl, dbl}[] []) -> ()  [unwired: 2 in, 2 out]
                    n356 = Wait (ms)(milliseconds to wait=1000) -> ()  [unwired: 1 out]
                    n357 = property on="XY图" class="XYGraph (严格)"("XScale.Minimum"=w431, "XScale.Maximum"=w430, "YScale.Minimum"=w431, "YScale.Maximum"=w430) -> ()  [unwired: 2 in, 2 out]
                    n358 = property on="XY图" class="XYGraph (严格)"("Value"=w435) -> ()  [unwired: 2 in, 2 out]
                  }
                }
              }
              frame #1 {
                n359 = local read "板子选择"() -> (w445:bool)
                n360 = local read "波形选择"() -> (w446:enum32{"斜坡", "正弦", "PWM波", "直流", "控制"})
                n361 = Boolean To (0,1)(Boolean=w445) -> (0, 1=w444:i16)
                n362 = case shown="\"斜坡\", 默认" w446 {
                  selector: w446 -> [w456 w469 w484 w500]
                  tunnel: [w463 w472 w487 w499] -> w442
                  tunnel: w444 -> [w455 w468 w483 w501]
                  frame "斜坡", Default {
                    w467 = 170
                    n363 = local read "通道D"() -> (w457:enum16{"DA0", "DA1", "DA01", ""})
                    n364 = local read "斜率k"() -> (w462:dbl)
                    n365 = local read "极值"() -> (w460:dbl)
                    n366 = local read "截距"() -> (w465:dbl)
                    n367 = call "浮点转字节数组.vi"("输入"=w460) -> ("数组，高字节在前"=w458:u8[])  [unwired: 3 in, 4 out]
                    n368 = call "浮点转字节数组.vi"("输入"=w462) -> ("数组，高字节在前"=w466:u8[])  [unwired: 3 in, 4 out]
                    n369 = call "浮点转字节数组.vi"("输入"=w465) -> ("数组，高字节在前"=w464:u8[])  [unwired: 3 in, 4 out]
                    n370 = Build Array (concatenate)(w467, w467, w455, w457, w456, w466, w464, w458, 0) -> (w461:u32[])
                    n371 = Byte Array To String(unsigned byte array=w461) -> (string=w463:string)
                    n372 = local write "发送区"(w463) -> ()
                  }
                  frame "正弦" {
                    w482 = 170
                    n373 = local read "通道S"() -> (w470:enum16{"DA0", "DA1", "DA01", ""})
                    n374 = local read "正弦角频率"() -> (w479:dbl)
                    n375 = local read "初相"() -> (w478:dbl)
                    n376 = local read "偏距"() -> (w474:dbl)
                    n377 = local read "振幅"() -> (w481:dbl)
                    n378 = call "浮点转字节数组.vi"("输入"=w481) -> ("数组，高字节在前"=w480:u8[])  [unwired: 3 in, 4 out]
                    n379 = call "浮点转字节数组.vi"("输入"=w479) -> ("数组，高字节在前"=w477:u8[])  [unwired: 3 in, 4 out]
                    n380 = call "浮点转字节数组.vi"("输入"=w478) -> ("数组，高字节在前"=w476:u8[])  [unwired: 3 in, 4 out]
                    n381 = call "浮点转字节数组.vi"("输入"=w474) -> ("数组，高字节在前"=w475:u8[])  [unwired: 3 in, 4 out]
                    n382 = Build Array (concatenate)(w482, w482, w468, w470, w469, w480, w477, w476, w475, 0) -> (w471:u32[])
                    n383 = Byte Array To String(unsigned byte array=w471) -> (string=w472:string)
                    n384 = local write "发送区"(w472) -> ()
                  }
                  frame "PWM波" {
                    w497 = 170
                    n385 = local read "通道P"() -> (w485:enum16{"DA0", "DA1", "DA01", ""})
                    n386 = local read "PWM波频率"() -> (w492:dbl)
                    n387 = local read "占空比"() -> (w490:dbl)
                    n388 = local read "高电压"() -> (w496:dbl)
                    n389 = local read "低电压"() -> (w494:dbl)
                    n390 = call "浮点转字节数组.vi"("输入"=w496) -> ("数组，高字节在前"=w495:u8[])  [unwired: 3 in, 4 out]
                    n391 = call "浮点转字节数组.vi"("输入"=w494) -> ("数组，高字节在前"=w493:u8[])  [unwired: 3 in, 4 out]
                    n392 = call "浮点转字节数组.vi"("输入"=w492) -> ("数组，高字节在前"=w491:u8[])  [unwired: 3 in, 4 out]
                    n393 = call "浮点转字节数组.vi"("输入"=w490) -> ("数组，高字节在前"=w489:u8[])  [unwired: 3 in, 4 out]
                    n394 = Build Array (concatenate)(w497, w497, w483, w485, w484, w495, w493, w491, w489, 0) -> (w486:u32[])
                    n395 = Byte Array To String(unsigned byte array=w486) -> (string=w487:string)
                    n396 = local write "发送区"(w487) -> ()
                  }
                  frame "直流" {
                    n397 = local read "自动测量"() -> (w498:bool)
                    n398 = case shown="真" w498 {
                      tunnel: w501 -> [_ w510]
                      tunnel: w500 -> [_ w507]
                      tunnel: ["\r\n" w503] -> w499
                      frame False {
                      }
                      frame True {
                        w508 = 2  # 通道
                        w509 = 170
                        n399 = local read "DA01"() -> (w506:dbl)
                        n400 = local read "DA01"() -> (w505:dbl)
                        n401 = call "浮点转字节数组.vi"("输入"=w506) -> ("数组，高字节在前"=w513:u8[])  [unwired: 3 in, 4 out]
                        n402 = call "浮点转字节数组.vi"("输入"=w505) -> ("数组，高字节在前"=w512:u8[])  [unwired: 3 in, 4 out]
                        n403 = Build Array (concatenate)(w509, w509, w510, w508, w507, w513, w512, 0) -> (w504:u32[])
                        n404 = Byte Array To String(unsigned byte array=w504) -> (string=w503:string)
                      }
                    }
                    n405 = local write "发送区"(w499) -> ()
                  }
                }
                n406 = local read "串口状态"() -> (w443:bool)
                n407 = case shown="真" w443 {
                  tunnel: w442 -> [_ w448]
                  frame False {
                    n408 = One Button Dialog(message="未连接平台！") -> ()  [unwired: 1 in, 1 out]
                  }
                  frame True {
                    n409 = local read "端口"() -> (w449:string)
                    n410 = Concatenate Strings(w448, "\r\n") -> (w454:string)
                    n411 = local read "TX"() -> (w452:dbl)
                    n412 = VISA Write(VISA resource name=w449, write buffer=w454) -> (return count=w453:u32)  [unwired: 1 in, 2 out]
                    n413 = Add(x=w453, y=w452) -> (x+y=w450:dbl)
                    n414 = local write "TX"(w450) -> ()
                  }
                }
              }
            }
          }
          event "自动测量": Value Change {
            n415 = event-data() -> ("NewVal"=w514:bool)  [unwired: 1 in, 5 out]
            n416 = case shown="真" w514 {
              frame False {
                w516 = 0
                n417 = property on="DA0" class="Slide (严格)"("DisabledEnum"=w516) -> ()  [unwired: 2 in, 2 out]
                n418 = property on="DA1" class="Slide (严格)"("DisabledEnum"=w516) -> ()  [unwired: 2 in, 2 out]
                n419 = property on="测量倒计时 S" class="DigNum (严格)"("DisabledEnum"=2) -> ()  [unwired: 2 in, 2 out]
              }
              frame True {
                w518 = 2
                n420 = property on="测量倒计时 S" class="DigNum (严格)"("DisabledEnum"=0) -> ()  [unwired: 2 in, 2 out]
                n421 = property on="DA0" class="Slide (严格)"("DisabledEnum"=w518) -> ()  [unwired: 2 in, 2 out]
                n422 = property on="DA1" class="Slide (严格)"("DisabledEnum"=w518) -> ()  [unwired: 2 in, 2 out]
              }
            }
          }
          event "断开连接时使波形归零": Value Change {
            n423 = event-data() -> ("NewVal"=w521:bool)  [unwired: 1 in, 5 out]
            n424 = case shown="假" w521 {
              frame False {
                n425 = One Button Dialog(message="断开连接后，平台将继续输出波形，但无法继续采集数据！") -> ()  [unwired: 1 in, 1 out]
              }
              frame True {
              }
            }
          }
          event "DA0": Value Change {
            w523 = u16 0 items=["0xAA"=170, "CH0"=0, "CH1"=1, "CH01"=2, "CARLIB"=85, "SWITCH"=86, "CONTROL"=87]
            w524 = u16 170 items=["0xAA"=170, "CH0"=0, "CH1"=1, "CH01"=2, "CARLIB"=85, "SWITCH"=86, "CONTROL"=87]
            n426 = event-data() -> ()  [unwired: 1 in, 6 out]
            n427 = local read "板子选择"() -> (w526:bool)
            n428 = local read "波形选择"() -> (w527:enum32{"斜坡", "正弦", "PWM波", "直流", "控制"})
            n429 = Boolean To (0,1)(Boolean=w526) -> (0, 1=w525:i16)
            n430 = local read "DA0"() -> (w536:dbl)
            n431 = local read "DA1"() -> (w535:dbl)
            n432 = call "浮点转字节数组.vi"("输入"=w536) -> ("数组，高字节在前"=w534:u8[])  [unwired: 3 in, 4 out]
            n433 = call "浮点转字节数组.vi"("输入"=w535) -> ("数组，高字节在前"=w533:u8[])  [unwired: 3 in, 4 out]
            n434 = Build Array (concatenate)(w524, w524, w525, w523, w527, w534, w533, 0) -> (w531:u32[])
            n435 = Byte Array To String(unsigned byte array=w531) -> (string=w529:string)
            n436 = local write "发送区"(w529) -> ()
            n437 = local read "串口状态"() -> (w530:bool)
            n438 = case shown="真" w530 {
              tunnel: w529 -> [_ w539]
              frame False {
                n439 = One Button Dialog(message="未连接平台！") -> ()  [unwired: 1 in, 1 out]
              }
              frame True {
                n440 = Concatenate Strings(w539, "\r\n") -> (w544:string)
                n441 = local read "端口"() -> (w538:string)
                n442 = local read "TX"() -> (w542:dbl)
                n443 = VISA Write(VISA resource name=w538, write buffer=w544) -> (return count=w543:u32)  [unwired: 1 in, 2 out]
                n444 = Add(x=w543, y=w542) -> (x+y=w540:dbl)
                n445 = local write "TX"(w540) -> ()
              }
            }
          }
          event "DA1": Value Change {
            w545 = u16 1 items=["0xAA"=170, "CH0"=0, "CH1"=1, "CH01"=2, "CARLIB"=85, "SWITCH"=86, "CONTROL"=87]
            w546 = u16 170 items=["0xAA"=170, "CH0"=0, "CH1"=1, "CH01"=2, "CARLIB"=85, "SWITCH"=86, "CONTROL"=87]
            n446 = event-data() -> ()  [unwired: 1 in, 6 out]
            n447 = local read "板子选择"() -> (w548:bool)
            n448 = local read "波形选择"() -> (w549:enum32{"斜坡", "正弦", "PWM波", "直流", "控制"})
            n449 = local read "DA0"() -> (w551:dbl)
            n450 = local read "DA1"() -> (w552:dbl)
            n451 = Boolean To (0,1)(Boolean=w548) -> (0, 1=w547:i16)
            n452 = call "浮点转字节数组.vi"("输入"=w551) -> ("数组，高字节在前"=w558:u8[])  [unwired: 3 in, 4 out]
            n453 = call "浮点转字节数组.vi"("输入"=w552) -> ("数组，高字节在前"=w557:u8[])  [unwired: 3 in, 4 out]
            n454 = Build Array (concatenate)(w546, w546, w547, w545, w549, w558, w557, 0) -> (w555:u32[])
            n455 = Byte Array To String(unsigned byte array=w555) -> (string=w554:string)
            n456 = local read "串口状态"() -> (w550:bool)
            n457 = case shown="真" w550 {
              tunnel: w554 -> [_ w561]
              frame False {
                n458 = One Button Dialog(message="未连接平台！") -> ()  [unwired: 1 in, 1 out]
              }
              frame True {
                n459 = local read "端口"() -> (w560:string)
                n460 = Concatenate Strings(w561, "\r\n") -> (w566:string)
                n461 = local read "TX"() -> (w564:dbl)
                n462 = VISA Write(VISA resource name=w560, write buffer=w566) -> (return count=w565:u32)  [unwired: 1 in, 2 out]
                n463 = Add(x=w565, y=w564) -> (x+y=w562:dbl)
                n464 = local write "TX"(w562) -> ()
              }
            }
          }
          event "DA01": Value Change {
            w567 = u16 2 items=["0xAA"=170, "CH0"=0, "CH1"=1, "CH01"=2, "CARLIB"=85, "SWITCH"=86, "CONTROL"=87]
            w568 = u16 170 items=["0xAA"=170, "CH0"=0, "CH1"=1, "CH01"=2, "CARLIB"=85, "SWITCH"=86, "CONTROL"=87]
            n465 = event-data() -> ()  [unwired: 1 in, 6 out]
            n466 = local read "板子选择"() -> (w578:bool)
            n467 = local read "波形选择"() -> (w574:enum32{"斜坡", "正弦", "PWM波", "直流", "控制"})
            n468 = Boolean To (0,1)(Boolean=w578) -> (0, 1=w577:i16)
            n469 = local read "DA01"() -> (w580:dbl)
            n470 = local read "DA01"() -> (w579:dbl)
            n471 = call "浮点转字节数组.vi"("输入"=w580) -> ("数组，高字节在前"=w583:u8[])  [unwired: 3 in, 4 out]
            n472 = call "浮点转字节数组.vi"("输入"=w579) -> ("数组，高字节在前"=w582:u8[])  [unwired: 3 in, 4 out]
            n473 = Build Array (concatenate)(w568, w568, w577, w567, w574, w583, w582, 0) -> (w576:u32[])
            n474 = local read "自动测量"() -> (w570:bool)
            n475 = Byte Array To String(unsigned byte array=w576) -> (string=w575:string)
            n476 = local read "串口状态"() -> (w572:bool)
            n477 = Not(x=w570) -> (.not. x?=w569:bool)
            n478 = And(x=w572, y=w569) -> (x .and. y?=w571:bool)
            n479 = case shown="真" w571 {
              tunnel: w575 -> [_ w585]
              frame False {
              }
              frame True {
                n480 = local read "端口"() -> (w589:string)
                n481 = Concatenate Strings(w585, "\r\n") -> (w584:string)
                n482 = local read "TX"() -> (w587:dbl)
                n483 = VISA Write(VISA resource name=w589, write buffer=w584) -> (return count=w588:u32)  [unwired: 1 in, 2 out]
                n484 = Add(x=w588, y=w587) -> (x+y=w586:dbl)
                n485 = local write "TX"(w586) -> ()
              }
            }
          }
          event "斜率角": Value Change {
            n486 = event-data() -> ("NewVal"=w594:dbl)  [unwired: 1 in, 5 out]
            n487 = expression code="(x/180.0)*pi" "角度转换至弧度"(w594) -> (w593:dbl)
            n488 = Tangent(1:w593) -> (0:w591:dbl)
            n489 = local write "斜率k"(w591) -> ()
          }
          event "正弦角频率": Value Change {
            n490 = event-data() -> ("NewVal"=w597:dbl)  [unwired: 1 in, 5 out]
            n491 = Multiply(x=2, y=3.141592653589793) -> (x*y=w596:dbl)
            n492 = Divide(x=w597, y=w596) -> (x/y=w595:dbl)
            n493 = local write "正弦频率"(w595) -> ()
          }
          event "高电压", "低电压": Value Change {
            n494 = event-data() -> ()  [unwired: 1 in, 6 out]
            n495 = local read "高电压"() -> (w603:dbl)
            n496 = local read "低电压"() -> (w602:dbl)
            n497 = Greater Or Equal?(x=w603, y=w602) -> (x >= y?=w604:bool)
            n498 = case shown="假" w604 {
              tunnel: w602 -> [w605 _]
              frame False {
                n499 = local write "高电压"(w605) -> ()
              }
              frame True {
              }
            }
          }
          event "控制方法": Value Change {
            n500 = event-data() -> ("NewVal"=w607:T2)  [unwired: 1 in, 5 out]
            n501 = case shown="\"PID控制\", 默认" w607 {
              frame "PID控制", Default {
                n502 = property on="KD" class="DigNum (严格)"("Visible"=TRUE) -> ()  [unwired: 2 in, 2 out]
              }
              frame "BangBang控制" {
                n503 = property on="KD" class="DigNum (严格)"("Visible"=FALSE) -> ()  [unwired: 2 in, 2 out]
              }
            }
          }
          event "发送控制数据": Mouse Up {
            w610 = u16 170 items=["0xAA"=170, "CH0"=0, "CH1"=1, "CH01"=2, "CARLIB"=85, "SWITCH"=86, "CONTROL"=87]
            w611 = u16 87 items=["0xAA"=170, "CH0"=0, "CH1"=1, "CH01"=2, "CARLIB"=85, "SWITCH"=86, "CONTROL"=87]
            n504 = event-data() -> ()  [unwired: 1 in, 8 out]
            n505 = local read "板子选择"() -> (w628:bool)
            n506 = Boolean To (0,1)(Boolean=w628) -> (0, 1=w629:i16)
            n507 = local read "外环KP/Bind"() -> (w621:dbl)
            n508 = local read "控制方法"() -> (w624:T2)
            n509 = local read "KP / HV"() -> (w620:dbl)
            n510 = local read "闭环对象"() -> (w617:enum16{"位移闭环", "功率闭环", "电流闭环", "力闭环"})
            n511 = local read "KI / LV"() -> (w619:dbl)
            n512 = local read "SetPoint"() -> (w623:dbl)
            n513 = local read "KD"() -> (w618:dbl)
            n514 = call "单精度浮点拆分.vi"("输入"=w623) -> ("小端数组"=w622:i32[])  [unwired: 3 in, 4 out]
            n515 = call "单精度浮点拆分.vi"("输入"=w621) -> ("小端数组"=w616:i32[])  [unwired: 3 in, 4 out]
            n516 = call "单精度浮点拆分.vi"("输入"=w620) -> ("小端数组"=w615:i32[])  [unwired: 3 in, 4 out]
            n517 = call "单精度浮点拆分.vi"("输入"=w619) -> ("小端数组"=w614:i32[])  [unwired: 3 in, 4 out]
            n518 = call "单精度浮点拆分.vi"("输入"=w618) -> ("小端数组"=w613:i32[])  [unwired: 3 in, 4 out]
            n519 = call "单精度浮点拆分.vi"("输入"=w617) -> ("小端数组"=w612:i32[])  [unwired: 3 in, 4 out]
            n520 = Build Array (concatenate)(w610, w610, w629, w611, w611, w624, w622, w616, w615, w614, w613, w612, 0) -> (w630:i32[])
            n521 = Byte Array To String(unsigned byte array=w630) -> (string=w626:string)
            n522 = local read "串口状态"() -> (w625:bool)
            n523 = case shown="真" w625 {
              tunnel: w626 -> [_ w634]
              frame False {
                n524 = One Button Dialog(message="未连接平台！") -> ()  [unwired: 1 in, 1 out]
              }
              frame True {
                n525 = Concatenate Strings(w634, "\r\n") -> (w639:string)
                n526 = local read "端口"() -> (w633:string)
                n527 = local read "TX"() -> (w637:dbl)
                n528 = VISA Write(VISA resource name=w633, write buffer=w639) -> (return count=w638:u32)  [unwired: 1 in, 2 out]
                n529 = Add(x=w638, y=w637) -> (x+y=w635:dbl)
                n530 = local write "TX"(w635) -> ()
              }
            }
          }
        }
      }
      frame "Exit" {
      }
    }
  }
  n531 = while {
    stop <- FALSE stop-if-true
    (unwired) 150
    n532 = local read "串口状态"() -> (w644:bool)
    n533 = Wait (ms) ("等待(ms)")(milliseconds to wait="接收间隔ms") -> ()  [unwired: 1 out]
    n534 = case shown="真" w644 {
      frame False {
      }
      frame True {
        n535 = local read "端口"() -> (w646:string)
        n536 = VISA Read(VISA resource name=w646, byte count=0) -> (VISA resource name out=w649:refnum<visa-resource-name>)  [unwired: 1 in, 3 out]
        n537 = property class="Serial Instr"(reference=w649) -> ("Bytes at Port"=w647:u32)  [unwired: 1 in, 2 out]
        n538 = property on="接收区" class="Str"("Text.Scroll Position"=inf) -> ()  [unwired: 2 in, 2 out]
        n539 = Greater Than 0?(x=w647) -> (x > 0?=w648:bool)
        n540 = case shown="真" w648 {
          tunnel: w646 -> [_ w666]
          tunnel: w647 -> [_ w665]
          frame False {
          }
          frame True {
            # "关闭解析减少不匹配\n引起的卡顿"
            n541 = local read "RX"() -> (w668:u64)
            n542 = VISA Read(VISA resource name=w666, byte count=w665) -> (read buffer=w651:string, return count=w667:u32)  [unwired: 1 in, 2 out]
            "接收区" <- w651
            n543 = Add(x=w667, y=w668) -> (x+y=w664:u64)
            "RX" <- w664
            n544 = disable-structure shown="禁用" {
              disable-tunnel: w664 -> [w675 _]
              frame Disabled {
                w674 = 20000
                # "定时清空接收区以保证不卡顿"
                n545 = Quotient & Remainder(x=w675, y=w674) -> (x-y*floor(x/y)=w671:u64)  [unwired: 1 out]
                n546 = Less?(x=w671, y=100) -> (x < y?=w670:bool)
                n547 = Greater?(x=w675, y=w674) -> (0:w673:bool)
                n548 = And(x=w673, y=w670) -> (x .and. y?=w672:bool)
                n549 = case shown="真" w672 {
                  frame False {
                  }
                  frame True {
                    n550 = property on="接收区" class="Str"("Value"="接收区\n") -> ()  [unwired: 2 in, 2 out]
                  }
                }
              }
              frame Enabled {
              }
            }
            n551 = local read "匹配剩余"() -> (w654:string)
            n552 = local read "调试模式"() -> (w653:bool)
            n553 = local read "接收间隔ms"() -> (w663:u16)
            n554 = Not(x=w653) -> (.not. x?=w652:bool)
            n555 = call "解析协议.vi"("新数据"=w651, "上次未匹配数据"=w654, "使能解析"=w652) -> ("其他数据簇"=w655:T7, "剩余未匹配数据"=→"匹配剩余":string, "传感数据组"=w657:T8, "解析成功"=w656:bool)  [unwired: 1 out]
            n556 = Array Size(array=w657) -> (size(s)=w662:i32)
            n557 = Divide(x=w663, y=w662) -> (x/y=w660:dbl)
            n558 = Divide(x=1000, y=w660) -> (x/y=→"实时采样率 Hz":dbl)
            n559 = case shown="真" w656 {
              tunnel: w657 -> [_ w701]
              tunnel: w657 -> [_ w695]
              tunnel: w655 -> [_ w700]
              frame False {
                "误码" <- TRUE
              }
              frame True {
                n560 = Index Array(array=w701) -> (element=w704:T9)  [unwired: 1 in]
                n561 = Unbundle(w700) -> ("温度"=→"温度 ℃":dbl, "湿度"=→"湿度 %":dbl, "CPU使用率"=→"CPU %":dbl)  [unwired: 2 out]
                n562 = Unbundle(w704) -> ("电流"=w685:dbl, "电压"=→"电压 V":dbl, "力"=w682:dbl, "激光"=→"位移 mm":dbl, "电阻"=→"电阻 R":dbl, "功率"=w679:dbl)
                n563 = Multiply(x=1000, y=w685) -> (x*y=→"电流 mA":dbl)
                n564 = call "调整采样率.vi"("目标采样率 Hz"="采样率 Hz", "输入"=w695) -> ("输出"=w693:T8)  [unwired: 3 in]
                n565 = Array Size(array=w693) -> (size(s)=w690:i32)
                n566 = Add(x="图表点数", y=w690) -> (x+y=w692:i32)
                n567 = Multiply(x=1000, y=w682) -> (x*y=→"力 mN":dbl)
                n568 = Divide(x=w682, y=9.8) -> (x/y=w709:dbl)
                n569 = local write "图表点数"(w692) -> ()
                n570 = Multiply(x=1000, y=w709) -> (x*y=w706:dbl)
                n571 = Absolute Value(x=w706) -> (abs(x)=→"质量 g":dbl)
                n572 = local read "能量 J"() -> (w687:dbl)
                n573 = case shown="真" "打开图表" {
                  tunnel: w693 -> [_ w717]
                  frame False {
                  }
                  frame True {
                    n574 = Bundle("X"="X", "Y"="Y") -> (w711:T10)  [unwired: 1 in]
                    n575 = call "XY图数据提取.vi"("XY对"=w711, "输入数据"=w717) -> ("提取后XY对数组"=w716:cluster{dbl, dbl}[])  [unwired: 3 in]
                    n576 = Insert Into Array(array="XY缓存", new element=w716) -> (w714:cluster{dbl, dbl}[])  [unwired: 1 in]
                    "XY图" <- w714
                    n577 = local write "XY缓存"(w714) -> ()
                    "波形图表" <- w717
                  }
                }
                n578 = Multiply(x=1000, y=w679) -> (x*y=→"功率 mW":dbl)
                n579 = Add(x=w687, y=w687) -> (x+y=→"能量 J":dbl)
                n580 = local write "误码"(FALSE) -> ()
              }
            }
          }
        }
      }
    }
  }
  n581 = timed-loop {
    timing: w2 -> [_]
    timing-out: [_] -> w1
    stop <- _ stop-if-true
    n582 = node-c288() -> ()  [unwired: 1 in, 1 out]
    n583 = local read "采样率 Hz"() -> (w721:u16)
    n584 = local read "图表点数"() -> (w722:i32)
    n585 = Reciprocal(x=w721) -> (1/x=w720:dbl)
    n586 = Get Date/Time In Seconds() -> (seconds since 1Jan1904=w724:timestamp)
    n587 = Multiply(x=w722, y=w720) -> (x*y=→"持续时间 S":dbl)
    n588 = Format Date/Time String(seconds (now)=w724) -> (date/time string=w723:string)  [unwired: 2 in]
    n589 = local write "系统时间"(w723) -> ()
    n590 = local read "定时开始"() -> (w718:bool)
    n591 = case shown="真" w718 {
      frame False {
      }
      frame True {
        n592 = local read "测量倒计时 S"() -> (w730:dbl)
        n593 = local read "定时结束"() -> (w727:dbl)
        n594 = call <vilib>:"High Resolution Relative Seconds.vi"() -> ("relative seconds"=w725:dbl)
        n595 = Greater?(x=w725, y=w727) -> (0:w726:bool)
        n596 = Subtract(x=w730, y=0.2) -> (x-y=w728:dbl)
        n597 = local write "测量倒计时 S"(w728) -> ()
        n598 = case shown="真" w726 {
          frame False {
          }
          frame True {
            n599 = local write "测量倒计时 S"(0.0) -> ()
            n600 = local read "板子选择"() -> (w732:bool)
            n601 = local write "定时开始"(FALSE) -> ()
            n602 = local read "端口"() -> (w733:string)
            n603 = local read "串口状态"() -> (w734:bool)
            n604 = call "清除波形.vi"("板子选择"=w732) -> ("输出字符串"=w731:string)
            n605 = case shown="真" w734 {
              tunnel: w731 -> [_ w743]
              tunnel: w733 -> [_ w739]
              frame False {
              }
              frame True {
                w737 = FALSE
                n606 = local read "断开连接时使波形归零"() -> (w738:bool)
                n607 = case shown="真" w738 {
                  tunnel: w743 -> [_ w752]
                  tunnel: [w745 w748] -> w741
                  tunnel: [errorcluster {"status"=FALSE, "code"=0, "source"=""} ("错误常量") w747] -> w740
                  tunnel: w739 -> [w745 w746]
                  frame False {
                  }
                  frame True {
                    n608 = local read "TX"() -> (w750:dbl)
                    n609 = VISA Write(VISA resource name=w746, write buffer=w752) -> (VISA resource name out=w748:refnum<visa-resource-name>, return count=w751:u32, error out=w747:errorcluster)  [unwired: 1 in]
                    n610 = Add(x=w751, y=w750) -> (x+y=w749:dbl)
                    n611 = local write "TX"(w749) -> ()
                  }
                }
                n612 = VISA Close(VISA resource name=w741, error in (no error)=w740) -> (error out=w742:errorcluster)
                n613 = local write "串口状态"(w737) -> ()
                n614 = local write "连接"(w737) -> ()
                n615 = call <vilib>:"Simple Error Handler.vi"("error in (no error)"=w742) -> ()  [unwired: 4 in, 5 out]
              }
            }
          }
        }
      }
    }
    n616 = node-c288() -> ()  [unwired: 1 in, 1 out]
  }
  n617 = node-c288(w1) -> ()  [unwired: 1 out]
